vi "Play.vi"() -> ()   [LabVIEW 2018]
uses:
  Downloads/Snake-master/Typedefs/State Machine.ctl
  Downloads/Snake-master/Globals/Keypress Global.vi
panel:
  in  "Stop":bool
  out "Your Score":i32 format="%#.0f"
  in  "Map":u32[][](array[colorbox])
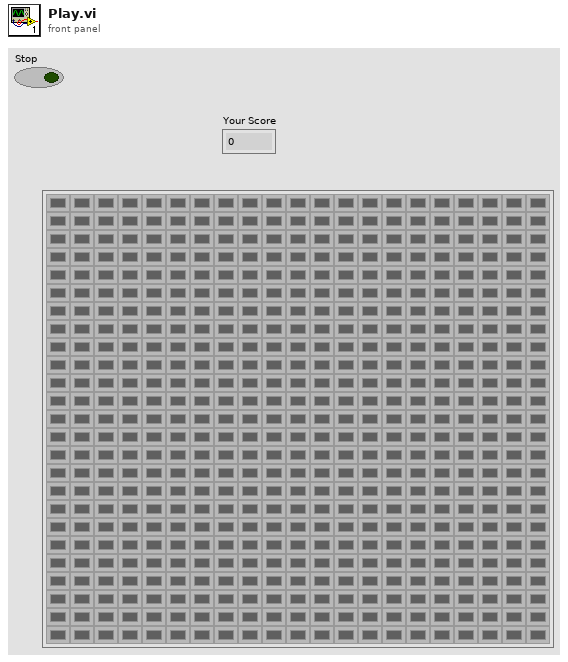
[diagram p1: front panel]
types:
  T1 = enum16{"Initialise", "Collision Check", "Grow Tail", "Move", "Wait", "Spawn Food", "Update", "Game Over"}
  T2 = typedef "State Machine.ctl" = enum16{"Initalize", "Collision Check", "Grow Tail", "Move", "Wait", "Spawn Food", "Update", "Game Over"}
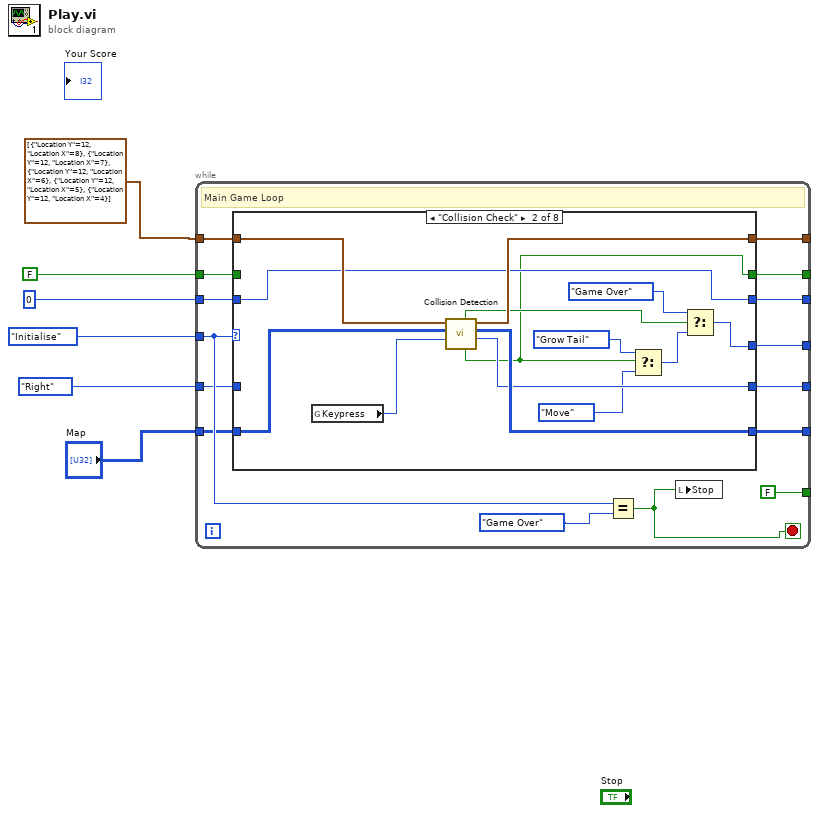
[diagram p0: block diagram]
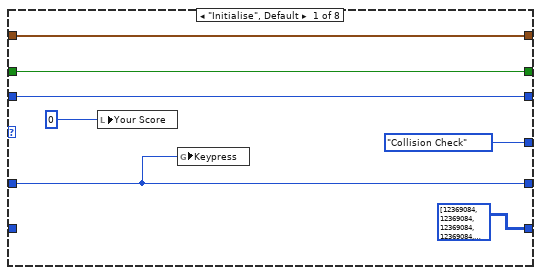
[diagram p2: hidden frame]
diagram:
  n1 = while {
    tunnel: cluster{"Location Y":i32, "Location X":i32}[] [{"Location Y"=12, "Location X"=8}, {"Location Y"=12, "Location X"=7}, {"Location Y"=12, "Location X"=6}, {"Location Y"=12, "Location X"=5}, {"Location Y"=12, "Location X"=4}] -> [w17]
    tunnel: T1."Initialise" -> [w20]
    tunnel: enum16{"Right", "Down", "Up", "Left"}."Right" ("KeyPress") -> [w19]
    tunnel: "Map" -> [w13]
    tunnel: FALSE -> [w18]
    tunnel: 0 -> [w16]
    tunnel: [FALSE] -> _
    tunnel: [w12] -> _
    tunnel: [w11] -> _
    tunnel: [w10] -> _
    tunnel: [w9] -> _
    tunnel: [w8] -> _
    tunnel: [w7] -> _
    stop <- w15 stop-if-true
    # "Main Game Loop"
    n2 = case shown="\"Collision Check\"" w20 {
      tunnel: w19 -> [w24 _ _ _ _ _ _ _]
      tunnel: w18 -> [w26 _ _ _ _ _ _ _]
      tunnel: w17 -> [w27 w42 _ _ _ _ _ _]
      tunnel: w16 -> [w25 w30 _ _ _ _ _ _]
      tunnel: [State_Machine."Collision Check" w36 _ _ _ _ _ _] -> w12
      tunnel: [w27 w39 _ _ _ _ _ _] -> w9
      tunnel: [w26 w29 _ _ _ _ _ _] -> w10
      tunnel: [w25 w30 _ _ _ _ _ _] -> w11
      tunnel: [w24 w37 _ _ _ _ _ _] -> w8
      tunnel: w13 -> [_ w41 _ _ _ _ _ _]
      tunnel: [u32[][] [[12369084, 12369084, 12369084, 12369084, 12369084, 12369084, 12369084, 12369084, 12369084, 12369084, 12369084, 12369084, 12369084, 12369084, 12369084, 12369084, 12369084, 12369084, 12369084, 12369084, 12369084, 12369084, 12369084, 12369084, 12369084], [12369084, 12369084, 12369084, 12369084, 12369084, 12369084, 12369084, 12369084, 12369084, 12369084, 12369084, 12369084, 12369084, 12369084, 12369084, 12369084, 12369084, 12369084, 12369084, 12369084, 12369084, 12369084, 12369084, 12369084, 12369084], [12369084, 12369084, 12369084, 12369084, 12369084, 12369084, 12369084, 12369084, 12369084, 12369084, 12369084, 12369084, 12369084, 12369084, 12369084, 12369084, 12369084, 12369084, 12369084, 12369084, 12369084, 12369084, 12369084, 12369084, 12369084], [12369084, 12369084, 12369084, 12369084, 12369084, 12369084, 12369084, 12369084, 12369084, 12369084, 12369084, 12369084, 12369084, 12369084, 12369084, 12369084, 12369084, 12369084, 12369084, 12369084, 12369084, 12369084, 12369084, 12369084, 12369084], [12369084, 12369084, 12369084, 12369084, 12369084, 12369084, 12369084, 12369084, 12369084, 12369084, 12369084, 12369084, 12369084, 12369084, 12369084, 12369084, 12369084, 12369084, 12369084, 12369084, 12369084, 12369084, 12369084, 12369084, 12369084], [12369084, 12369084, 12369084, 12369084, 12369084, 12369084, 12369084, 12369084, 12369084, 12369084, 12369084, 12369084, 12369084, 12369084, 12369084, 12369084, 12369084, 12369084, 12369084, 12369084, 12369084, 12369084, 12369084, 12369084, 12369084], [12369084, 12369084, 12369084, 12369084, 12369084, 12369084, 12369084, 12369084, 12369084, 12369084, 12369084, 12369084, 12369084, 12369084, 12369084, 12369084, 12369084, 12369084, 12369084, 12369084, 12369084, 12369084, 12369084, 12369084, 12369084], [12369084, 12369084, 12369084, 12369084, 12369084, 12369084, 12369084, 12369084, 12369084, 12369084, 12369084, 12369084, 12369084, 12369084, 12369084, 12369084, 12369084, 12369084, 12369084, 12369084, 12369084, 12369084, 12369084, 12369084, 12369084], [12369084, 12369084, 12369084, 12369084, 12369084, 12369084, 12369084, 12369084, 12369084, 12369084, 12369084, 12369084, 12369084, 12369084, 12369084, 12369084, 12369084, 12369084, 12369084, 12369084, 12369084, 12369084, 12369084, 12369084, 12369084], [12369084, 12369084, 12369084, 12369084, 12369084, 12369084, 12369084, 12369084, 12369084, 12369084, 12369084, 12369084, 12369084, 12369084, 12369084, 12369084, 12369084, 12369084, 12369084, 12369084, 12369084, 12369084, 12369084, 12369084, 12369084], [12369084, 12369084, 12369084, 12369084, 12369084, 12369084, 12369084, 12369084, 12369084, 12369084, 12369084, 12369084, 12369084, 12369084, 12369084, 12369084, 12369084, 12369084, 12369084, 12369084, 12369084, 12369084, 12369084, 12369084, 12369084], [12369084, 12369084, 12369084, 12369084, 12369084, 12369084, 12369084, 12369084, 12369084, 12369084, 12369084, 12369084, 12369084, 12369084, 12369084, 12369084, 12369084, 12369084, 12369084, 12369084, 12369084, 12369084, 12369084, 12369084, 12369084], [12369084, 12369084, 12369084, 12369084, 16740721, 16740721, 16740721, 16740721, 16711680, 12369084, 12369084, 12369084, 12369084, 12369084, 12369084, 12369084, 12369084, 12369084, 12369084, 12369084, 12369084, 12369084, 12369084, 12369084, 12369084], [12369084, 12369084, 12369084, 12369084, 12369084, 12369084, 12369084, 12369084, 12369084, 12369084, 12369084, 12369084, 12369084, 12369084, 12369084, 12369084, 12369084, 12369084, 12369084, 12369084, 12369084, 12369084, 12369084, 12369084, 12369084], [12369084, 12369084, 12369084, 12369084, 12369084, 12369084, 12369084, 12369084, 12369084, 12369084, 12369084, 12369084, 12369084, 12369084, 12369084, 12369084, 12369084, 12369084, 12369084, 12369084, 12369084, 12369084, 12369084, 12369084, 12369084], [12369084, 12369084, 12369084, 12369084, 12369084, 12369084, 12369084, 12369084, 12369084, 12369084, 12369084, 12369084, 12369084, 12369084, 12369084, 12369084, 12369084, 12369084, 12369084, 12369084, 12369084, 12369084, 12369084, 12369084, 12369084], [12369084, 12369084, 12369084, 12369084, 12369084, 12369084, 12369084, 12369084, 12369084, 12369084, 12369084, 12369084, 12369084, 12369084, 12369084, 12369084, 12369084, 12369084, 12369084, 12369084, 12369084, 12369084, 12369084, 12369084, 12369084], [12369084, 12369084, 12369084, 12369084, 12369084, 12369084, 12369084, 12369084, 12369084, 12369084, 12369084, 12369084, 12369084, 12369084, 12369084, 12369084, 12369084, 12369084, 12369084, 12369084, 12369084, 12369084, 12369084, 12369084, 12369084], [12369084, 12369084, 12369084, 12369084, 12369084, 12369084, 12369084, 12369084, 12369084, 12369084, 12369084, 12369084, 12369084, 12369084, 12369084, 12369084, 12369084, 12369084, 12369084, 12369084, 12369084, 12369084, 12369084, 12369084, 12369084], [12369084, 12369084, 12369084, 12369084, 12369084, 12369084, 12369084, 12369084, 12369084, 12369084, 12369084, 12369084, 12369084, 12369084, 12369084, 12369084, 12369084, 12369084, 12369084, 12369084, 12369084, 12369084, 12369084, 12369084, 12369084], [12369084, 12369084, 12369084, 12369084, 12369084, 12369084, 12369084, 12369084, 12369084, 12369084, 12369084, 12369084, 12369084, 12369084, 12369084, 12369084, 12369084, 12369084, 12369084, 12369084, 12369084, 12369084, 12369084, 12369084, 12369084], [12369084, 12369084, 12369084, 12369084, 12369084, 12369084, 12369084, 12369084, 12369084, 12369084, 12369084, 12369084, 12369084, 12369084, 12369084, 12369084, 12369084, 12369084, 12369084, 12369084, 12369084, 12369084, 12369084, 12369084, 12369084], [12369084, 12369084, 12369084, 12369084, 12369084, 12369084, 12369084, 12369084, 12369084, 12369084, 12369084, 12369084, 12369084, 12369084, 12369084, 12369084, 12369084, 12369084, 12369084, 12369084, 12369084, 12369084, 12369084, 12369084, 12369084], [12369084, 12369084, 12369084, 12369084, 12369084, 12369084, 12369084, 12369084, 12369084, 12369084, 12369084, 12369084, 12369084, 12369084, 12369084, 12369084, 12369084, 12369084, 12369084, 12369084, 12369084, 12369084, 12369084, 12369084, 12369084], [12369084, 12369084, 12369084, 12369084, 12369084, 12369084, 12369084, 12369084, 12369084, 12369084, 12369084, 12369084, 12369084, 12369084, 12369084, 12369084, 12369084, 12369084, 12369084, 12369084, 12369084, 12369084, 12369084, 12369084, 12369084]] ("Map") w38 _ _ _ _ _ _] -> w7
      frame "Initialise", Default {
        n3 = local write "Your Score"(0) -> ()
        n4 = global write "Keypress Global.vi" "Keypress"(w24) -> ()
      }
      frame "Collision Check" {
        n5 = global read "Keypress Global.vi" "Keypress"() -> (w40:enum16{"Right", "Down", "Up", "Left"})
        n6 = call "Collision Detection.vi"("Keypress In"=w40, "Map In"=w41, "Locations In"=w42) -> ("Keypress Out"=w37:enum16{"Right", "Down", "Up", "Left"}, "Map Out"=w38:u32[][], "Locations Out"=w39:cluster{"Location Y":i32, "Location X":i32}[], "Collision?"=w29:bool, "Game Over?"=w31:bool)  [unwired: 4 in]
        n7 = Select(t=State_Machine."Grow Tail", s=w29, f=State_Machine."Move") -> (s? t:f=w35:T2)
        n8 = Select(t=State_Machine."Game Over", s=w31, f=w35) -> (s? t:f=w36:T2)
      }
      frame "Grow Tail" {
      }
      frame "Move" {
      }
      frame "Wait" {
      }
      frame "Spawn Food" {
      }
      frame "Update" {
      }
      frame "Game Over" {
      }
    }
    n9 = Equal?(x=w20, y=State_Machine."Game Over") -> (x = y?=w15:bool)
    n10 = local write "Stop"(w15) -> ()
  }
